vi "Weather Parse Test.vi"() -> ()   [LabVIEW 2020, in "CDM-Config.lvlib"] (continued)
                 ]\n                }\n            }\n        },\n        {\n            \"id\": \"https://api.weather.gov/alerts/urn:oid:2.49.0.1.840.0.415ec53db9f1e26240148abfa70e4c09e2d74678.012.1\",\n            \"type\": \"Feature\",\n            \"geometry\": null,\n            \"properties\": {\n                \"@id\": \"https://api.weather.gov/alerts/urn:oid:2.49.0.1.840.0.415ec53db9f1e26240148abfa70e4c09e2d74678.012.1\",\n                \"@type\": \"wx:Alert\",\n                \"id\": \"urn:oid:2.49.0.1.840.0.415ec53db9f1e26240148abfa70e4c09e2d74678.012.1\",\n                \"areaDesc\": \"Icy Cape to Cape Suckling out to 15 NM\",\n                \"geocode\": {\n                    \"SAME\": [\n                        \"058652\"\n                    ],\n                    \"UGC\": [\n                        \"PKZ652\"\n                    ]\n                },\n                \"affectedZones\": [\n                    \"https://api.weather.gov/zones/forecast/PKZ652\"\n                ],\n                \"references\": [],\n                \"sent\": \"2025-12-03T02:44:00-09:00\",\n                \"effective\": \"2025-12-03T02:44:00-09:00\",\n                \"onset\": \"2025-12-03T02:00:00-09:00\",\n                \"expires\": \"2025-12-03T20:45:00-09:00\",\n                \"ends\": \"2025-12-04T05:00:00-09:00\",\n                \"status\": \"Actual\",\n                \"messageType\": \"Alert\",\n                \"category\": \"Met\",\n                \"severity\": \"Minor\",\n                \"certainty\": \"Likely\",\n                \"urgency\": \"Expected\",\n                \"event\": \"Small Craft Advisory\",\n                \"sender\": \"w-nws.webmaster@noaa.gov\",\n                \"senderName\": \"NWS Juneau AK\",\n                \"headline\": \"Small Craft Advisory issued December 3 at 2:44AM AKST until December 4 at 5:00AM AKST by NWS Juneau AK\",\n                \"description\": \"Southeast Alaska Coastal Waters from Dixon Entrance to\\nCape Suckling out 100 NM\\n\\nWind forecasts reflect the predominant speed and direction\\nexpected. Seas forecasts represent the average of the highest\\none-third of the combined windwave and swell height.\\n\\n.TODAY...E wind 25 kt diminishing to 15 kt in the afternoon. Seas\\n12 ft. Rain.\\n.TONIGHT...Light winds becoming W 10 kt late. Seas 9 ft. SW\\nswell.\\n.THU...Light winds. Seas 8 ft. SW swell.\\n.THU NIGHT...E wind 10 kt. Seas 7 ft. SW swell.\\n.FRI...E wind 20 kt. Seas 7 ft.\\n.SAT...E gale to 35 kt. Seas 12 ft.\\n.SUN...E gale to 35 kt. Seas 15 ft.\",\n                \"instruction\": null,\n                \"response\": \"Avoid\",\n                \"parameters\": {\n                    \"AWIPSidentifier\": [\n                        \"CWFAEG\"\n                    ],\n                    \"WMOidentifier\": [\n                        \"FZAK52 PAJK 031144\"\n                    ],\n                    \"NWSheadline\": [\n                        \"SMALL CRAFT ADVISORY THROUGH LATE TONIGHT\"\n                    ],\n                    \"BLOCKCHANNEL\": [\n                        \"EAS\",\n                        \"NWEM\",\n                        \"CMAS\"\n                    ],\n                    \"VTEC\": [\n                        \"/O.NEW.PAJK.SC.Y.8602.251203T1100Z-251204T1400Z/\"\n                    ],\n                    \"eventEndingTime\": [\n                        \"2025-12-04T05:00:00-09:00\"\n                    ]\n                },\n                \"scope\": \"Public\",\n                \"code\": \"IPAWSv1.0\",\n                \"language\": \"en-US\",\n                \"web\": \"http://www.weather.gov\",\n                \"eventCode\": {\n                    \"SAME\": [\n                        \"NWS\"\n                    ],\n                    \"NationalWeatherService\": [\n                        \"SCY\"\n                    ]\n                }\n            }\n        },\n        {\n            \"id\": \"https://api.weather.gov/alerts/urn:oid:2.49.0.1.840.0.415ec53db9f1e26240148abfa70e4c09e2d74678.005.1\",\n            \"type\": \"Feature\",\n            \"geometry\": null,\n            \"properties\": {\n                \"@id\": \"https://api.weather.gov/alerts/urn:oid:2.49.0.1.840.0.415ec53db9f1e26240148abfa70e4c09e2d74678.005.1\",\n                \"@type\": \"wx:Alert\",\n                \"id\": \"urn:oid:2.49.0.1.840.0.415ec53db9f1e26240148abfa70e4c09e2d74678.005.1\",\n                \"areaDesc\": \"Cape Decision to Cape Edgecumbe from 15 to 80 NM\",\n                \"geocode\": {\n                    \"SAME\": [\n                        \"058662\"\n                    ],\n                    \"UGC\": [\n                        \"PKZ662\"\n                    ]\n                },\n                \"affectedZones\": [\n                    \"https://api.weather.gov/zones/forecast/PKZ662\"\n                ],\n                \"references\": [],\n                \"sent\": \"2025-12-03T02:44:00-09:00\",\n                \"effective\": \"2025-12-03T02:44:00-09:00\",\n                \"onset\": \"2025-12-03T02:00:00-09:00\",\n                \"expires\": \"2025-12-03T20:45:00-09:00\",\n                \"ends\": \"2025-12-04T05:00:00-09:00\",\n                \"status\": \"Actual\",\n                \"messageType\": \"Alert\",\n                \"category\": \"Met\",\n                \"severity\": \"Minor\",\n                \"certainty\": \"Likely\",\n                \"urgency\": \"Expected\",\n                \"event\": \"Small Craft Advisory\",\n                \"sender\": \"w-nws.webmaster@noaa.gov\",\n                \"senderName\": \"NWS Juneau AK\",\n                \"headline\": \"Small Craft Advisory issued December 3 at 2:44AM AKST until December 4 at 5:00AM AKST by NWS Juneau AK\",\n                \"description\": \"Southeast Alaska Coastal Waters from Dixon Entrance to\\nCape Suckling out 100 NM\\n\\nWind forecasts reflect the predominant speed and direction\\nexpected. Seas forecasts represent the average of the highest\\none-third of the combined windwave and swell height.\\n\\n.TODAY...S wind 20 kt becoming W in the afternoon. Seas 11 ft.\\n.TONIGHT...W wind 15 kt. Seas 10 ft.\\n.THU...W wind 10 kt becoming S in the afternoon. Seas 8 ft.\\n.THU NIGHT...SE wind 20 kt. Seas 9 ft.\\n.FRI...W wind 25 kt. Seas 14 ft.\\n.SAT...S wind 30 kt. Seas 16 ft.\\n.SUN...S gale to 35 kt. Seas 21 ft.\",\n                \"instruction\": null,\n                \"response\": \"Avoid\",\n                \"parameters\": {\n                    \"AWIPSidentifier\": [\n                        \"CWFAEG\"\n                    ],\n                    \"WMOidentifier\": [\n                        \"FZAK52 PAJK 031144\"\n                    ],\n                    \"NWSheadline\": [\n                        \"SMALL CRAFT ADVISORY THROUGH LATE TONIGHT\"\n                    ],\n                    \"BLOCKCHANNEL\": [\n                        \"EAS\",\n                        \"NWEM\",\n                        \"CMAS\"\n                    ],\n                    \"VTEC\": [\n                        \"/O.NEW.PAJK.SC.Y.8595.251203T1100Z-251204T1400Z/\"\n                    ],\n                    \"eventEndingTime\": [\n                        \"2025-12-04T05:00:00-09:00\"\n                    ]\n                },\n                \"scope\": \"Public\",\n                \"code\": \"IPAWSv1.0\",\n                \"language\": \"en-US\",\n                \"web\": \"http://www.weather.gov\",\n                \"eventCode\": {\n                    \"SAME\": [\n                        \"NWS\"\n                    ],\n                    \"NationalWeatherService\": [\n                        \"SCY\"\n                    ]\n                }\n            }\n        },\n        {\n            \"id\": \"https://api.weather.gov/alerts/urn:oid:2.49.0.1.840.0.415ec53db9f1e26240148abfa70e4c09e2d74678.009.1\",\n            \"type\": \"Feature\",\n            \"geometry\": null,\n            \"properties\": {\n                \"@id\": \"https://api.weather.gov/alerts/urn:oid:2.49.0.1.840.0.415ec53db9f1e26240148abfa70e4c09e2d74678.009.1\",\n                \"@type\": \"wx:Alert\",\n                \"id\": \"urn:oid:2.49.0.1.840.0.415ec53db9f1e26240148abfa70e4c09e2d74678.009.1\",\n                \"areaDesc\": \"Cape Spencer to Cape Fairweather from 15 to 85 NM\",\n                \"geocode\": {\n                    \"SAME\": [\n                        \"058664\"\n                    ],\n                    \"UGC\": [\n                        \"PKZ664\"\n                    ]\n                },\n                \"affectedZones\": [\n                    \"https://api.weather.gov/zones/forecast/PKZ664\"\n                ],\n                \"references\": [],\n                \"sent\": \"2025-12-03T02:44:00-09:00\",\n                \"effective\": \"2025-12-03T02:44:00-09:00\",\n                \"onset\": \"2025-12-03T02:00:00-09:00\",\n                \"expires\": \"2025-12-03T20:45:00-09:00\",\n                \"ends\": \"2025-12-04T05:00:00-09:00\",\n                \"status\": \"Actual\",\n                \"messageType\": \"Alert\",\n                \"category\": \"Met\",\n                \"severity\": \"Minor\",\n                \"certainty\": \"Likely\",\n                \"urgency\": \"Expected\",\n                \"event\": \"Small Craft Advisory\",\n                \"sender\": \"w-nws.webmaster@noaa.gov\",\n                \"senderName\": \"NWS Juneau AK\",\n                \"headline\": \"Small Craft Advisory issued December 3 at 2:44AM AKST until December 4 at 5:00AM AKST by NWS Juneau AK\",\n                \"description\": \"Southeast Alaska Coastal Waters from Dixon Entrance to\\nCape Suckling out 100 NM\\n\\nWind forecasts reflect the predominant speed and direction\\nexpected. Seas forecasts represent the average of the highest\\none-third of the combined windwave and swell height.\\n\\n.TODAY...S wind 25 kt becoming SW 15 kt in the afternoon. Seas\\n11 ft. SW swell.\\n.TONIGHT...W wind 20 kt. Seas 10 ft.\\n.THU...W wind 10 kt. Seas 9 ft.\\n.THU NIGHT...SE wind 20 kt. Seas 8 ft.\\n.FRI...SW wind 25 kt. Seas 9 ft.\\n.SAT...S gale to 35 kt. Seas 15 ft.\\n.SUN...S gale to 35 kt. Seas 18 ft.\",\n                \"instruction\": null,\n                \"response\": \"Avoid\",\n                \"parameters\": {\n                    \"AWIPSidentifier\": [\n                        \"CWFAEG\"\n                    ],\n                    \"WMOidentifier\": [\n                        \"FZAK52 PAJK 031144\"\n                    ],\n                    \"NWSheadline\": [\n                        \"SMALL CRAFT ADVISORY THROUGH LATE TONIGHT\"\n                    ],\n                    \"BLOCKCHANNEL\": [\n                        \"EAS\",\n                        \"NWEM\",\n                        \"CMAS\"\n                    ],\n                    \"VTEC\": [\n                        \"/O.NEW.PAJK.SC.Y.8599.251203T1100Z-251204T1400Z/\"\n                    ],\n                    \"eventEndingTime\": [\n                        \"2025-12-04T05:00:00-09:00\"\n                    ]\n                },\n                \"scope\": \"Public\",\n                \"code\": \"IPAWSv1.0\",\n                \"language\": \"en-US\",\n                \"web\": \"http://www.weather.gov\",\n                \"eventCode\": {\n                    \"SAME\": [\n                        \"NWS\"\n                    ],\n                    \"NationalWeatherService\": [\n                        \"SCY\"\n                    ]\n                }\n            }\n        },\n        {\n            \"id\": \"https://api.weather.gov/alerts/urn:oid:2.49.0.1.840.0.415ec53db9f1e26240148abfa70e4c09e2d74678.007.1\",\n            \"type\": \"Feature\",\n            \"geometry\": null,\n            \"properties\": {\n                \"@id\": \"https://api.weather.gov/alerts/urn:oid:2.49.0.1.840.0.415ec53db9f1e26240148abfa70e4c09e2d74678.007.1\",\n                \"@type\": \"wx:Alert\",\n                \"id\": \"urn:oid:2.49.0.1.840.0.415ec53db9f1e26240148abfa70e4c09e2d74678.007.1\",\n                \"areaDesc\": \"Cape Edgecumbe to Cape Spencer from 15 to 80 NM\",\n                \"geocode\": {\n                    \"SAME\": [\n                        \"058663\"\n                    ],\n                    \"UGC\": [\n                        \"PKZ663\"\n                    ]\n                },\n                \"affectedZones\": [\n                    \"https://api.weather.gov/zones/forecast/PKZ663\"\n                ],\n                \"references\": [],\n                \"sent\": \"2025-12-03T02:44:00-09:00\",\n                \"effective\": \"2025-12-03T02:44:00-09:00\",\n                \"onset\": \"2025-12-03T02:00:00-09:00\",\n                \"expires\": \"2025-12-03T20:45:00-09:00\",\n                \"ends\": \"2025-12-04T05:00:00-09:00\",\n                \"status\": \"Actual\",\n                \"messageType\": \"Alert\",\n                \"category\": \"Met\",\n                \"severity\": \"Minor\",\n                \"certainty\": \"Likely\",\n                \"urgency\": \"Expected\",\n                \"event\": \"Small Craft Advisory\",\n                \"sender\": \"w-nws.webmaster@noaa.gov\",\n                \"senderName\": \"NWS Juneau AK\",\n                \"headline\": \"Small Craft Advisory issued December 3 at 2:44AM AKST until December 4 at 5:00AM AKST by NWS Juneau AK\",\n                \"description\": \"Southeast Alaska Coastal Waters from Dixon Entrance to\\nCape Suckling out 100 NM\\n\\nWind forecasts reflect the predominant speed and direction\\nexpected. Seas forecasts represent the average of the highest\\none-third of the combined windwave and swell height.\\n\\n.TODAY...S wind 20 kt becoming W in the afternoon. Seas 11 ft.\\n.TONIGHT...W wind 20 kt. Seas 10 ft.\\n.THU...SW wind 10 kt. Seas 9 ft.\\n.THU NIGHT...SE wind 20 kt. Seas 9 ft.\\n.FRI...SW wind 20 kt. Seas 10 ft.\\n.SAT...S wind 30 kt. Seas 14 ft.\\n.SUN...S wind 30 kt. Seas 20 ft.\",\n                \"instruction\": null,\n                \"response\": \"Avoid\",\n                \"parameters\": {\n                    \"AWIPSidentifier\": [\n                        \"CWFAEG\"\n                    ],\n                    \"WMOidentifier\": [\n                        \"FZAK52 PAJK 031144\"\n                    ],\n                    \"NWSheadline\": [\n                        \"SMALL CRAFT ADVISORY THROUGH LATE TONIGHT\"\n                    ],\n                    \"BLOCKCHANNEL\": [\n                        \"EAS\",\n                        \"NWEM\",\n                        \"CMAS\"\n                    ],\n                    \"VTEC\": [\n                        \"/O.NEW.PAJK.SC.Y.8597.251203T1100Z-251204T1400Z/\"\n                    ],\n                    \"eventEndingTime\": [\n                        \"2025-12-04T05:00:00-09:00\"\n                    ]\n                },\n                \"scope\": \"Public\",\n                \"code\": \"IPAWSv1.0\",\n                \"language\": \"en-US\",\n                \"web\": \"http://www.weather.gov\",\n                \"eventCode\": {\n                    \"SAME\": [\n                        \"NWS\"\n                    ],\n                    \"NationalWeatherService\": [\n                        \"SCY\"\n                    ]\n                }\n            }\n        },\n        {\n            \"id\": \"https://api.weather.gov/alerts/urn:oid:2.49.0.1.840.0.415ec53db9f1e26240148abfa70e4c09e2d74678.008.1\",\n            \"type\": \"Feature\",\n            \"geometry\": null,\n            \"properties\": {\n                \"@id\": \"https://api.weather.gov/alerts/urn:oid:2.49.0.1.840.0.415ec53db9f1e26240148abfa70e4c09e2d74678.008.1\",\n                \"@type\": \"wx:Alert\",\n                \"id\": \"urn:oid:2.49.0.1.840.0.415ec53db9f1e26240148abfa70e4c09e2d74678.008.1\",\n                \"areaDesc\": \"Cape Spencer to Cape Fairweather out to 15 NM\",\n                \"geocode\": {\n                    \"SAME\": [\n                        \"058644\"\n                    ],\n                    \"UGC\": [\n                        \"PKZ644\"\n                    ]\n                },\n                \"affectedZones\": [\n                    \"https://api.weather.gov/zones/forecast/PKZ644\"\n                ],\n                \"references\": [],\n                \"sent\": \"2025-12-03T02:44:00-09:00\",\n                \"effective\": \"2025-12-03T02:44:00-09:00\",\n                \"onset\": \"2025-12-03T02:00:00-09:00\",\n                \"expires\": \"2025-12-03T20:45:00-09:00\",\n                \"ends\": \"2025-12-04T05:00:00-09:00\",\n                \"status\": \"Actual\",\n                \"messageType\": \"Alert\",\n                \"category\": \"Met\",\n                \"severity\": \"Minor\",\n                \"certainty\": \"Likely\",\n                \"urgency\": \"Expected\",\n                \"event\": \"Small Craft Advisory\",\n                \"sender\": \"w-nws.webmaster@noaa.gov\",\n                \"senderName\": \"NWS Juneau AK\",\n                \"headline\": \"Small Craft Advisory issued December 3 at 2:44AM AKST until December 4 at 5:00AM AKST by NWS Juneau AK\",\n                \"description\": \"Southeast Alaska Coastal Waters from Dixon Entrance to\\nCape Suckling out 100 NM\\n\\nWind forecasts reflect the predominant speed and direction\\nexpected. Seas forecasts represent the average of the highest\\none-third of the combined windwave and swell height.\\n\\n.TODAY...E wind 25 kt becoming SE 15 kt in the afternoon. Seas\\n11 ft. Rain.\\n.TONIGHT...W wind 15 kt. Seas 10 ft.\\n.THU...W wind 10 kt. Seas 9 ft.\\n.THU NIGHT...E wind 15 kt. Seas 8 ft.\\n.FRI...NE wind 25 kt. Seas 9 ft.\\n.SAT...S gale to 35 kt. Seas 14 ft.\\n.SUN...SE gale to 35 kt. Seas 17 ft.\",\n                \"instruction\": null,\n                \"response\": \"Avoid\",\n                \"parameters\": {\n                    \"AWIPSidentifier\": [\n                        \"CWFAEG\"\n                    ],\n                    \"WMOidentifier\": [\n                        \"FZAK52 PAJK 031144\"\n                    ],\n                    \"NWSheadline\": [\n                        \"SMALL CRAFT ADVISORY THROUGH LATE TONIGHT\"\n                    ],\n                    \"BLOCKCHANNEL\": [\n                        \"EAS\",\n                        \"NWEM\",\n                        \"CMAS\"\n                    ],\n                    \"VTEC\": [\n                        \"/O.NEW.PAJK.SC.Y.8598.251203T1100Z-251204T1400Z/\"\n                    ],\n                    \"eventEndingTime\": [\n                        \"2025-12-04T05:00:00-09:00\"\n                    ]\n                },\n                \"scope\": \"Public\",\n                \"code\": \"IPAWSv1.0\",\n                \"language\": \"en-US\",\n                \"web\": \"http://www.weather.gov\",\n                \"eventCode\": {\n                    \"SAME\": [\n                        \"NWS\"\n                    ],\n                    \"NationalWeatherService\": [\n                        \"SCY\"\n                    ]\n                }\n            }\n        },\n        {\n            \"id\": \"https://api.weather.gov/alerts/urn:oid:2.49.0.1.840.0.415ec53db9f1e26240148abfa70e4c09e2d74678.006.1\",\n            \"type\": \"Feature\",\n            \"geometry\": null,\n            \"properties\": {\n                \"@id\": \"https://api.weather.gov/alerts/urn:oid:2.49.0.1.840.0.415ec53db9f1e26240148abfa70e4c09e2d74678.006.1\",\n                \"@type\": \"wx:Alert\",\n                \"id\": \"urn:oid:2.49.0.1.840.0.415ec53db9f1e26240148abfa70e4c09e2d74678.006.1\",\n                \"areaDesc\": \"Cape Edgecumbe to Cape Spencer out to 15 NM\",\n                \"geocode\": {\n                    \"SAME\": [\n                        \"058643\"\n                    ],\n                    \"UGC\": [\n                        \"PKZ643\"\n                    ]\n                },\n                \"affectedZones\": [\n                    \"https://api.weather.gov/zones/forecast/PKZ643\"\n                ],\n                \"references\": [],\n                \"sent\": \"2025-12-03T02:44:00-09:00\",\n                \"effective\": \"2025-12-03T02:44:00-09:00\",\n                \"onset\": \"2025-12-03T02:00:00-09:00\",\n                \"expires\": \"2025-12-03T20:45:00-09:00\",\n                \"ends\": \"2025-12-04T05:00:00-09:00\",\n                \"status\": \"Actual\",\n                \"messageType\": \"Alert\",\n                \"category\": \"Met\",\n                \"severity\": \"Minor\",\n                \"certainty\": \"Likely\",\n                \"urgency\": \"Expected\",\n                \"event\": \"Small Craft Advisory\",\n                \"sender\": \"w-nws.webmaster@noaa.gov\",\n                \"senderName\": \"NWS Juneau AK\",\n                \"headline\": \"Small Craft Advisory issued December 3 at 2:44AM AKST until December 4 at 5:00AM AKST by NWS Juneau AK\",\n                \"description\": \"Southeast Alaska Coastal Waters from Dixon Entrance to\\nCape Suckling out 100 NM\\n\\nWind forecasts reflect the predominant speed and direction\\nexpected. Seas forecasts represent the average of the highest\\none-third of the combined windwave and swell height.\\n\\n.TODAY...SE wind 25 kt becoming SW 15 kt in the afternoon. Seas\\n11 ft. Rain early in the morning.\\n.TONIGHT...W wind 15 kt. Seas 10 ft.\\n.THU...SW wind 10 kt. Seas 9 ft.\\n.THU NIGHT...E wind 15 kt. Seas 8 ft.\\n.FRI...NE wind 20 kt. Seas 10 ft.\\n.SAT...S wind 30 kt. Seas 13 ft.\\n.SUN...S wind 30 kt. Seas 17 ft.\",\n                \"instruction\": null,\n                \"response\": \"Avoid\",\n                \"parameters\": {\n                    \"AWIPSidentifier\": [\n                        \"CWFAEG\"\n                    ],\n                    \"WMOidentifier\": [\n                        \"FZAK52 PAJK 031144\"\n                    ],\n                    \"NWSheadline\": [\n                        \"SMALL CRAFT ADVISORY THROUGH LATE TONIGHT\"\n                    ],\n                    \"BLOCKCHANNEL\": [\n                        \"EAS\",\n                        \"NWEM\",\n                        \"CMAS\"\n                    ],\n                    \"VTEC\": [\n                        \"/O.NEW.PAJK.SC.Y.8596.251203T1100Z-251204T1400Z/\"\n                    ],\n                    \"eventEndingTime\": [\n                        \"2025-12-04T05:00:00-09:00\"\n                    ]\n                },\n                \"scope\": \"Public\",\n                \"code\": \"IPAWSv1.0\",\n                \"language\": \"en-US\",\n                \"web\": \"http://www.weather.gov\",\n                \"eventCode\": {\n                    \"SAME\": [\n                        \"NWS\"\n                    ],\n                    \"NationalWeatherService\": [\n                        \"SCY\"\n                    ]\n                }\n            }\n        },\n        {\n            \"id\": \"https://api.weather.gov/alerts/urn:oid:2.49.0.1.840.0.415ec53db9f1e26240148abfa70e4c09e2d74678.010.1\",\n            \"type\": \"Feature\",\n            \"geometry\": null,\n            \"properties\": {\n                \"@id\": \"https://api.weather.gov/alerts/urn:oid:2.49.0.1.840.0.415ec53db9f1e26240148abfa70e4c09e2d74678.010.1\",\n                \"@type\": \"wx:Alert\",\n                \"id\": \"urn:oid:2.49.0.1.840.0.415ec53db9f1e26240148abfa70e4c09e2d74678.010.1\",\n                \"areaDesc\": \"Cape Fairweather to Icy Cape out to 15 NM\",\n                \"geocode\": {\n                    \"SAME\": [\n                        \"058651\"\n                    ],\n                    \"UGC\": [\n                        \"PKZ651\"\n                    ]\n                },\n                \"affectedZones\": [\n                    \"https://api.weather.gov/zones/forecast/PKZ651\"\n                ],\n                \"references\": [],\n                \"sent\": \"2025-12-03T02:44:00-09:00\",\n                \"effective\": \"2025-12-03T02:44:00-09:00\",\n                \"onset\": \"2025-12-03T02:00:00-09:00\",\n                \"expires\": \"2025-12-03T20:45:00-09:00\",\n                \"ends\": \"2025-12-04T05:00:00-09:00\",\n                \"status\": \"Actual\",\n                \"messageType\": \"Alert\",\n                \"category\": \"Met\",\n                \"severity\": \"Minor\",\n                \"certainty\": \"Likely\",\n                \"urgency\": \"Expected\",\n                \"event\": \"Small Craft Advisory\",\n                \"sender\": \"w-nws.webmaster@noaa.gov\",\n                \"senderName\": \"NWS Juneau AK\",\n                \"headline\": \"Small Craft Advisory issued December 3 at 2:44AM AKST until December 4 at 5:00AM AKST by NWS Juneau AK\",\n                \"description\": \"Southeast Alaska Coastal Waters from Dixon Entrance to\\nCape Suckling out 100 NM\\n\\nWind forecasts reflect the predominant speed and direction\\nexpected. Seas forecasts represent the average of the highest\\none-third of the combined windwave and swell height.\\n\\n.TODAY...SE wind 25 kt becoming SW 15 kt in the afternoon. Seas\\n11 ft. Rain.\\n.TONIGHT...W wind 10 kt. Seas 10 ft.\\n.THU...Light winds becoming E 10 kt in the afternoon. Seas\\n8 ft. SW swell.\\n.THU NIGHT...E wind 10 kt. Seas 7 ft. SW swell.\\n.FRI...E wind 25 kt. Seas 9 ft.\\n.SAT...E gale to 35 kt. Seas 14 ft.\\n.SUN...E gale to 35 kt. Seas 16 ft.\",\n                \"instruction\": null,\n                \"response\": \"Avoid\",\n                \"parameters\": {\n                    \"AWIPSidentifier\": [\n                        \"CWFAEG\"\n                    ],\n                    \"WMOidentifier\": [\n                        \"FZAK52 PAJK 031144\"\n                    ],\n                    \"NWSheadline\": [\n                        \"SMALL CRAFT ADVISORY THROUGH LATE TONIGHT\"\n                    ],\n                    \"BLOCKCHANNEL\": [\n                        \"EAS\",\n                        \"NWEM\",\n                        \"CMAS\"\n                    ],\n                    \"VTEC\": [\n                        \"/O.NEW.PAJK.SC.Y.8600.251203T1100Z-251204T1400Z/\"\n                    ],\n                    \"eventEndingTime\": [\n                        \"2025-12-04T05:00:00-09:00\"\n                    ]\n                },\n                \"scope\": \"Public\",\n                \"code\": \"IPAWSv1.0\",\n                \"language\": \"en-US\",\n                \"web\": \"http://www.weather.gov\",\n                \"eventCode\": {\n                    \"SAME\": [\n                        \"NWS\"\n                    ],\n                    \"NationalWeatherService\": [\n                        \"SCY\"\n                    ]\n                }\n            }\n        },\n        {\n            \"id\": \"https://api.weather.gov/alerts/urn:oid:2.49.0.1.840.0.415ec53db9f1e26240148abfa70e4c09e2d74678.002.1\",\n            \"type\": \"Feature\",\n            \"geometry\": null,\n            \"properties\": {\n                \"@id\": \"https://api.weather.gov/alerts/urn:oid:2.49.0.1.840.0.415ec53db9f1e26240148abfa70e4c09e2d74678.002.1\",\n                \"@type\": \"wx:Alert\",\n                \"id\": \"urn:oid:2.49.0.1.840.0.415ec53db9f1e26240148abfa70e4c09e2d74678.002.1\",\n                \"areaDesc\": \"Dixon Entrance to Cape Decision out to 15 NM\",\n                \"geocode\": {\n                    \"SAME\": [\n                        \"058641\"\n                    ],\n                    \"UGC\": [\n                        \"PKZ641\"\n                    ]\n                },\n                \"affectedZones\": [\n                    \"https://api.weather.gov/zones/forecast/PKZ641\"\n                ],\n                \"references\": [],\n                \"sent\": \"2025-12-03T02:44:00-09:00\",\n                \"effective\": \"2025-12-03T02:44:00-09:00\",\n                \"onset\": \"2025-12-03T02:00:00-09:00\",\n                \"expires\": \"2025-12-03T20:45:00-09:00\",\n                \"ends\": \"2025-12-04T05:00:00-09:00\",\n                \"status\": \"Actual\",\n                \"messageType\": \"Alert\",\n                \"category\": \"Met\",\n                \"severity\": \"Minor\",\n                \"certainty\": \"Likely\",\n                \"urgency\": \"Expected\",\n                \"event\": \"Small Craft Advisory\",\n                \"sender\": \"w-nws.webmaster@noaa.gov\",\n                \"senderName\": \"NWS Juneau AK\",\n                \"headline\": \"Small Craft Advisory issued December 3 at 2:44AM AKST until December 4 at 5:00AM AKST by NWS Juneau AK\",\n                \"description\": \"Southeast Alaska Coastal Waters from Dixon Entrance to\\nCape Suckling out 100 NM\\n\\nWind forecasts reflect the predominant speed and direction\\nexpected. Seas forecasts represent the average of the highest\\none-third of the combined windwave and swell height.\\n\\n.TODAY...SE wind 25 kt becoming W 15 kt in the afternoon. Seas\\n11 ft. Rain early in the morning.\\n.TONIGHT...W wind 10 kt. Seas 10 ft.\\n.THU...W wind 10 kt becoming SE in the afternoon. Seas 8 ft.\\nSW swell.\\n.THU NIGHT...SE wind 20 kt. Seas 9 ft. Rain.\\n.FRI...W wind 25 kt. Seas 15 ft.\\n.SAT...S wind 30 kt. Seas 15 ft.\\n.SUN...S gale to 40 kt. Seas 20 ft.\",\n                \"instruction\": null,\n                \"response\": \"Avoid\",\n                \"parameters\": {\n                    \"AWIPSidentifier\": [\n                        \"CWFAEG\"\n                    ],\n                    \"WMOidentifier\": [\n                        \"FZAK52 PAJK 031144\"\n                    ],\n                    \"NWSheadline\": [\n                        \"SMALL CRAFT ADVISORY THROUGH LATE TONIGHT\"\n                    ],\n                    \"BLOCKCHANNEL\": [\n                        \"EAS\",\n                        \"NWEM\",\n                        \"CMAS\"\n                    ],\n                    \"VTEC\": [\n                        \"/O.NEW.PAJK.SC.Y.8592.251203T1100Z-251204T1400Z/\"\n                    ],\n                    \"eventEndingTime\": [\n                        \"2025-12-04T05:00:00-09:00\"\n                    ]\n                },\n                \"scope\": \"Public\",\n                \"code\": \"IPAWSv1.0\",\n                \"language\": \"en-US\",\n                \"web\": \"http://www.weather.gov\",\n                \"eventCode\": {\n                    \"SAME\": [\n                        \"NWS\"\n                    ],\n                    \"NationalWeatherService\": [\n                        \"SCY\"\n                    ]\n                }\n            }\n        },\n        {\n            \"id\": \"https://api.weather.gov/alerts/urn:oid:2.49.0.1.840.0.415ec53db9f1e26240148abfa70e4c09e2d74678.004.1\",\n            \"type\": \"Feature\",\n            \"geometry\": null,\n            \"properties\": {\n                \"@id\": \"https://api.weather.gov/alerts/urn:oid:2.49.0.1.840.0.415ec53db9f1e26240148abfa70e4c09e2d74678.004.1\",\n                \"@type\": \"wx:Alert\",\n                \"id\": \"urn:oid:2.49.0.1.840.0.415ec53db9f1e26240148abfa70e4c09e2d74678.004.1\",\n                \"areaDesc\": \"Cape Decision to Cape Edgecumbe out to 15 NM\",\n                \"geocode\": {\n                    \"SAME\": [\n                        \"058642\"\n                    ],\n                    \"UGC\": [\n                        \"PKZ642\"\n                    ]\n                },\n                \"affectedZones\": [\n                    \"https://api.weather.gov/zones/forecast/PKZ642\"\n                ],\n                \"references\": [],\n                \"sent\": \"2025-12-03T02:44:00-09:00\",\n                \"effective\": \"2025-12-03T02:44:00-09:00\",\n                \"onset\": \"2025-12-03T02:00:00-09:00\",\n                \"expires\": \"2025-12-03T20:45:00-09:00\",\n                \"ends\": \"2025-12-04T05:00:00-09:00\",\n                \"status\": \"Actual\",\n                \"messageType\": \"Alert\",\n                \"category\": \"Met\",\n                \"severity\": \"Minor\",\n                \"certainty\": \"Likely\",\n                \"urgency\": \"Expected\",\n                \"event\": \"Small Craft Advisory\",\n                \"sender\": \"w-nws.webmaster@noaa.gov\",\n                \"senderName\": \"NWS Juneau AK\",\n                \"headline\": \"Small Craft Advisory issued December 3 at 2:44AM AKST until December 4 at 5:00AM AKST by NWS Juneau AK\",\n                \"description\": \"Southeast Alaska Coastal Waters from Dixon Entrance to\\nCape Suckling out 100 NM\\n\\nWind forecasts reflect the predominant speed and direction\\nexpected. Seas forecasts represent the average of the highest\\none-third of the combined windwave and swell height.\\n\\n.TODAY...SE wind 25 kt becoming W 15 kt in the afternoon. Seas\\n11 ft. Rain early in the morning.\\n.TONIGHT...W wind 15 kt. Seas 10 ft.\\n.THU...W wind 10 kt becoming S in the afternoon. Seas 8 ft.\\n.THU NIGHT...E wind 20 kt. Seas 9 ft.\\n.FRI...W wind 20 kt. Seas 13 ft.\\n.SAT...S wind 30 kt. Seas 15 ft.\\n.SUN...S gale to 35 kt. Seas 20 ft.\",\n                \"instruction\": null,\n                \"response\": \"Avoid\",\n                \"parameters\": {\n                    \"AWIPSidentifier\": [\n                        \"CWFAEG\"\n                    ],\n                    \"WMOidentifier\": [\n                        \"FZAK52 PAJK 031144\"\n                    ],\n                    \"NWSheadline\": [\n                        \"SMALL CRAFT ADVISORY THROUGH LATE TONIGHT\"\n                    ],\n                    \"BLOCKCHANNEL\": [\n                        \"EAS\",\n                        \"NWEM\",\n                        \"CMAS\"\n                    ],\n                    \"VTEC\": [\n                        \"/O.NEW.PAJK.SC.Y.8594.251203T1100Z-251204T1400Z/\"\n                    ],\n                    \"eventEndingTime\": [\n                        \"2025-12-04T05:00:00-09:00\"\n                    ]\n                },\n                \"scope\": \"Public\",\n                \"code\": \"IPAWSv1.0\",\n                \"language\": \"en-US\",\n                \"web\": \"http://www.weather.gov\",\n                \"eventCode\": {\n                    \"SAME\": [\n                        \"NWS\"\n                    ],\n                    \"NationalWeatherService\": [\n                        \"SCY\"\n                    ]\n                }\n            }\n        },\n        {\n            \"id\": \"https://api.weather.gov/alerts/urn:oid:2.49.0.1.840.0.415ec53db9f1e26240148abfa70e4c09e2d74678.003.1\",\n            \"type\": \"Feature\",\n            \"geometry\": null,\n            \"properties\": {\n                \"@id\": \"https://api.weather.gov/alerts/urn:oid:2.49.0.1.840.0.415ec53db9f1e26240148abfa70e4c09e2d74678.003.1\",\n                \"@type\": \"wx:Alert\",\n                \"id\": \"urn:oid:2.49.0.1.840.0.415ec53db9f1e26240148abfa70e4c09e2d74678.003.1\",\n                \"areaDesc\": \"Dixon Entrance to Cape Decision from 15 to 90 NM\",\n                \"geocode\": {\n                    \"SAME\": [\n                        \"058661\"\n                    ],\n                    \"UGC\": [\n                        \"PKZ661\"\n                    ]\n                },\n                \"affectedZones\": [\n                    \"https://api.weather.gov/zones/forecast/PKZ661\"\n                ],\n                \"references\": [],\n                \"sent\": \"2025-12-03T02:44:00-09:00\",\n                \"effective\": \"2025-12-03T02:44:00-09:00\",\n                \"onset\": \"2025-12-03T02:00:00-09:00\",\n                \"expires\": \"2025-12-03T20:45:00-09:00\",\n                \"ends\": \"2025-12-04T05:00:00-09:00\",\n                \"status\": \"Actual\",\n                \"messageType\": \"Alert\",\n                \"category\": \"Met\",\n                \"severity\": \"Minor\",\n                \"certainty\": \"Likely\",\n                \"urgency\": \"Expected\",\n                \"event\": \"Small Craft Advisory\",\n                \"sender\": \"w-nws.webmaster@noaa.gov\",\n                \"senderName\": \"NWS Juneau AK\",\n                \"headline\": \"Small Craft Advisory issued December 3 at 2:44AM AKST until December 4 at 5:00AM AKST by NWS Juneau AK\",\n                \"description\": \"Southeast Alaska Coastal Waters from Dixon Entrance to\\nCape Suckling out 100 NM\\n\\nWind forecasts reflect the predominant speed and direction\\nexpected. Seas forecasts represent the average of the highest\\none-third of the combined windwave and swell height.\\n\\n.TODAY...SW wind 20 kt becoming W in the afternoon. Seas 11 ft.\\nRain early in the morning.\\n.TONIGHT...W wind 15 kt. Seas 10 ft.\\n.THU...W wind 10 kt becoming SE in the afternoon. Seas 8 ft.\\nSW swell.\\n.THU NIGHT...SE wind 25 kt. Seas 9 ft. Rain.\\n.FRI...W wind 25 kt. Seas 17 ft.\\n.SAT...SW wind 30 kt. Seas 16 ft.\\n.SUN...SW gale to 35 kt. Seas 22 ft.\",\n                \"instruction\": null,\n                \"response\": \"Avoid\",\n                \"parameters\": {\n                    \"AWIPSidentifier\": [\n                        \"CWFAEG\"\n                    ],\n                    \"WMOidentifier\": [\n                        \"FZAK52 PAJK 031144\"\n                    ],\n                    \"NWSheadline\": [\n                        \"SMALL CRAFT ADVISORY THROUGH LATE TONIGHT\"\n                    ],\n                    \"BLOCKCHANNEL\": [\n                        \"EAS\",\n                        \"NWEM\",\n                        \"CMAS\"\n                    ],\n                    \"VTEC\": [\n                        \"/O.NEW.PAJK.SC.Y.8593.251203T1100Z-251204T1400Z/\"\n                    ],\n                    \"eventEndingTime\": [\n                        \"2025-12-04T05:00:00-09:00\"\n                    ]\n                },\n                \"scope\": \"Public\",\n                \"code\": \"IPAWSv1.0\",\n                \"language\": \"en-US\",\n                \"web\": \"http://www.weather.gov\",\n                \"eventCode\": {\n                    \"SAME\": [\n                        \"NWS\"\n                    ],\n                    \"NationalWeatherService\": [\n                        \"SCY\"\n                    ]\n                }\n            }\n        },\n        {\n            \"id\": \"https://api.weather.gov/alerts/urn:oid:2.49.0.1.840.0.415ec53db9f1e26240148abfa70e4c09e2d74678.013.1\",\n            \"type\": \"Feature\",\n            \"geometry\": null,\n            \"properties\": {\n                \"@id\": \"https://api.weather.gov/alerts/urn:oid:2.49.0.1.840.0.415ec53db9f1e26240148abfa70e4c09e2d74678.013.1\",\n                \"@type\": \"wx:Alert\",\n                \"id\": \"urn:oid:2.49.0.1.840.0.415ec53db9f1e26240148abfa70e4c09e2d74678.013.1\",\n                \"areaDesc\": \"Icy Cape to Cape Suckling from 15 to 80 NM\",\n                \"geocode\": {\n                    \"SAME\": [\n                        \"058672\"\n                    ],\n                    \"UGC\": [\n                        \"PKZ672\"\n                    ]\n                },\n                \"affectedZones\": [\n                    \"https://api.weather.gov/zones/forecast/PKZ672\"\n                ],\n                \"references\": [],\n                \"sent\": \"2025-12-03T02:44:00-09:00\",\n                \"effective\": \"2025-12-03T02:44:00-09:00\",\n                \"onset\": \"2025-12-03T02:00:00-09:00\",\n                \"expires\": \"2025-12-03T20:45:00-09:00\",\n                \"ends\": \"2025-12-04T05:00:00-09:00\",\n                \"status\": \"Actual\",\n                \"messageType\": \"Alert\",\n                \"category\": \"Met\",\n                \"severity\": \"Minor\",\n                \"certainty\": \"Likely\",\n                \"urgency\": \"Expected\",\n                \"event\": \"Small Craft Advisory\",\n                \"sender\": \"w-nws.webmaster@noaa.gov\",\n                \"senderName\": \"NWS Juneau AK\",\n                \"headline\": \"Small Craft Advisory issued December 3 at 2:44AM AKST until December 4 at 5:00AM AKST by NWS Juneau AK\",\n                \"description\": \"Southeast Alaska Coastal Waters from Dixon Entrance to\\nCape Suckling out 100 NM\\n\\nWind forecasts reflect the predominant speed and direction\\nexpected. Seas forecasts represent the average of the highest\\none-third of the combined windwave and swell height.\\n\\n.TODAY...E wind 25 kt becoming SW 15 kt in the afternoon. Seas\\n12 ft.\\n.TONIGHT...W wind 15 kt. Seas 10 ft.\\n.THU...SW wind 10 kt. Seas 8 ft. SW swell.\\n.THU NIGHT...E wind 10 kt. Seas 8 ft.\\n.FRI...S wind 20 kt. Seas 8 ft.\\n.SAT...SE wind 30 kt. Seas 13 ft.\\n.SUN...SE wind 30 kt. Seas 16 ft.\",\n                \"instruction\": null,\n                \"response\": \"Avoid\",\n                \"parameters\": {\n                    \"AWIPSidentifier\": [\n                        \"CWFAEG\"\n                    ],\n                    \"WMOidentifier\": [\n                        \"FZAK52 PAJK 031144\"\n                    ],\n                    \"NWSheadline\": [\n                        \"SMALL CRAFT ADVISORY THROUGH LATE TONIGHT\"\n                    ],\n                    \"BLOCKCHANNEL\": [\n                        \"EAS\",\n                        \"NWEM\",\n                        \"CMAS\"\n                    ],\n                    \"VTEC\": [\n                        \"/O.NEW.PAJK.SC.Y.8603.251203T1100Z-251204T1400Z/\"\n                    ],\n                    \"eventEndingTime\": [\n                        \"2025-12-04T05:00:00-09:00\"\n                    ]\n                },\n                \"scope\": \"Public\",\n                \"code\": \"IPAWSv1.0\",\n                \"language\": \"en-US\",\n                \"web\": \"http://www.weather.gov\",\n                \"eventCode\": {\n                    \"SAME\": [\n                        \"NWS\"\n                    ],\n                    \"NationalWeatherService\": [\n                        \"SCY\"\n                    ]\n                }\n            }\n        },\n        {\n            \"id\": \"https://api.weather.gov/alerts/urn:oid:2.49.0.1.840.0.415ec53db9f1e26240148abfa70e4c09e2d74678.011.1\",\n            \"type\": \"Feature\",\n            \"geometry\": null,\n            \"properties\": {\n                \"@id\": \"https://api.weather.gov/alerts/urn:oid:2.49.0.1.840.0.415ec53db9f1e26240148abfa70e4c09e2d74678.011.1\",\n                \"@type\": \"wx:Alert\",\n                \"id\": \"urn:oid:2.49.0.1.840.0.415ec53db9f1e26240148abfa70e4c09e2d74678.011.1\",\n                \"areaDesc\": \"Cape Fairweather to Icy Cape from 15 to 80 NM\",\n                \"geocode\": {\n                    \"SAME\": [\n                        \"058671\"\n                    ],\n                    \"UGC\": [\n                        \"PKZ671\"\n                    ]\n                },\n                \"affectedZones\": [\n                    \"https://api.weather.gov/zones/forecast/PKZ671\"\n                ],\n                \"references\": [],\n                \"sent\": \"2025-12-03T02:44:00-09:00\",\n                \"effective\": \"2025-12-03T02:44:00-09:00\",\n                \"onset\": \"2025-12-03T02:00:00-09:00\",\n                \"expires\": \"2025-12-03T20:45:00-09:00\",\n                \"ends\": \"2025-12-04T05:00:00-09:00\",\n                \"status\": \"Actual\",\n                \"messageType\": \"Alert\",\n                \"category\": \"Met\",\n                \"severity\": \"Minor\",\n                \"certainty\": \"Likely\",\n                \"urgency\": \"Expected\",\n                \"event\": \"Small Craft Advisory\",\n                \"sender\": \"w-nws.webmaster@noaa.gov\",\n                \"senderName\": \"NWS Juneau AK\",\n                \"headline\": \"Small Craft Advisory issued December 3 at 2:44AM AKST until December 4 at 5:00AM AKST by NWS Juneau AK\",\n                \"description\": \"Southeast Alaska Coastal Waters from Dixon Entrance to\\nCape Suckling out 100 NM\\n\\nWind forecasts reflect the predominant speed and direction\\nexpected. Seas forecasts represent the average of the highest\\none-third of the combined windwave and swell height.\\n\\n.TODAY...S wind 25 kt becoming SW 15 kt in the afternoon. Seas\\n11 ft. SW swell. Rain early in the morning.\\n.TONIGHT...W wind 15 kt. Seas 10 ft.\\n.THU...SW wind 10 kt. Seas 9 ft.\\n.THU NIGHT...E wind 15 kt. Seas 8 ft.\\n.FRI...S wind 25 kt. Seas 9 ft.\\n.SAT...S gale to 35 kt. Seas 14 ft.\\n.SUN...SE gale to 35 kt. Seas 17 ft.\",\n                \"instruction\": null,\n                \"response\": \"Avoid\",\n                \"parameters\": {\n                    \"AWIPSidentifier\": [\n                        \"CWFAEG\"\n                    ],\n                    \"WMOidentifier\": [\n                        \"FZAK52 PAJK 031144\"\n                    ],\n                    \"NWSheadline\": [\n                        \"SMALL CRAFT ADVISORY THROUGH LATE TONIGHT\"\n                    ],\n                    \"BLOCKCHANNEL\": [\n                        \"EAS\",\n                        \"NWEM\",\n                        \"CMAS\"\n                    ],\n                    \"VTEC\": [\n                        \"/O.NEW.PAJK.SC.Y.8601.251203T1100Z-251204T1400Z/\"\n                    ],\n                    \"eventEndingTime\": [\n                        \"2025-12-04T05:00:00-09:00\"\n                    ]\n                },\n                \"scope\": \"Public\",\n                \"code\": \"IPAWSv1.0\",\n                \"language\": \"en-US\",\n                \"web\": \"http://www.weather.gov\",\n                \"eventCode\": {\n                    \"SAME\": [\n                        \"NWS\"\n                    ],\n                    \"NationalWeatherService\": [\n                        \"SCY\"\n                    ]\n                }\n            }\n        },\n        {\n            \"id\": \"https://api.weather.gov/alerts/urn:oid:2.49.0.1.840.0.94e4e19bc8eeb6087cc59420c6880e7d952ab5fe.006.1\",\n            \"type\": \"Feature\",\n            \"geometry\": null,\n            \"properties\": {\n                \"@id\": \"https://api.weather.gov/alerts/urn:oid:2.49.0.1.840.0.94e4e19bc8eeb6087cc59420c6880e7d952ab5fe.006.1\",\n                \"@type\": \"wx:Alert\",\n                \"id\": \"urn:oid:2.49.0.1.840.0.94e4e19bc8eeb6087cc59420c6880e7d952ab5fe.006.1\",\n                \"areaDesc\": \"Cross Sound\",\n                \"geocode\": {\n                    \"SAME\": [\n                        \"058022\"\n                    ],\n                    \"UGC\": [\n                        \"PKZ022\"\n                    ]\n                },\n                \"affectedZones\": [\n                    \"https://api.weather.gov/zones/forecast/PKZ022\"\n                ],\n                \"references\": [],\n                \"sent\": \"2025-12-03T02:44:00-09:00\",\n                \"effective\": \"2025-12-03T02:44:00-09:00\",\n                \"onset\": \"2025-12-03T02:00:00-09:00\",\n                \"expires\": \"2025-12-03T18:45:00-09:00\",\n                \"ends\": \"2025-12-04T05:00:00-09:00\",\n                \"status\": \"Actual\",\n                \"messageType\": \"Alert\",\n                \"category\": \"Met\",\n                \"severity\": \"Minor\",\n                \"certainty\": \"Likely\",\n                \"urgency\": \"Expected\",\n                \"event\": \"Small Craft Advisory\",\n                \"sender\": \"w-nws.webmaster@noaa.gov\",\n                \"senderName\": \"NWS Juneau AK\",\n                \"headline\": \"Small Craft Advisory issued December 3 at 2:44AM AKST until December 4 at 5:00AM AKST by NWS Juneau AK\",\n                \"description\": \"Southeast Alaska Inside Waters from Dixon Entrance to Skagway\\n\\nWind forecasts reflect the predominant speed and direction\\nexpected. Sea forecasts represent the average of the highest\\none-third of the combined windwave and swell height.\\n\\n.TODAY...E wind 15 kt becoming SW in the afternoon. Seas 9 ft.\\nRain.\\n.TONIGHT...SW wind 20 kt. Seas 8 ft. S swell. Rain in the\\nevening.\\n.THU...SW wind 10 kt. Seas 8 ft. Rain in the afternoon.\\n.THU NIGHT...NE wind 10 kt. Seas 7 ft. Rain.\\n.FRI...NE wind 15 kt. Seas 7 ft.\\n.SAT...S wind 25 kt. Seas 10 ft.\\n.SUN...E wind 30 kt. Seas 12 ft.\",\n                \"instruction\": null,\n                \"response\": \"Avoid\",\n                \"parameters\": {\n                    \"AWIPSidentifier\": [\n                        \"CWFAJK\"\n                    ],\n                    \"WMOidentifier\": [\n                        \"FZAK51 PAJK 031144\"\n                    ],\n                    \"NWSheadline\": [\n                        \"SMALL CRAFT ADVISORY THROUGH LATE TONIGHT\"\n                    ],\n                    \"BLOCKCHANNEL\": [\n                        \"EAS\",\n                        \"NWEM\",\n                        \"CMAS\"\n                    ],\n                    \"VTEC\": [\n                        \"/O.NEW.PAJK.SC.Y.7964.251203T1100Z-251204T1400Z/\"\n                    ],\n                    \"eventEndingTime\": [\n                        \"2025-12-04T05:00:00-09:00\"\n                    ]\n                },\n                \"scope\": \"Public\",\n                \"code\": \"IPAWSv1.0\",\n                \"language\": \"en-US\",\n                \"web\": \"http://www.weather.gov\",\n                \"eventCode\": {\n                    \"SAME\": [\n                        \"NWS\"\n                    ],\n                    \"NationalWeatherService\": [\n                        \"SCY\"\n                    ]\n                }\n            }\n        },\n        {\n            \"id\": \"https://api.weather.gov/alerts/urn:oid:2.49.0.1.840.0.4ff5fe1b1d40c5518c7c751190066b30fc728126.001.1\",\n            \"type\": \"Feature\",\n            \"geometry\": null,\n            \"properties\": {\n                \"@id\": \"https://api.weather.gov/alerts/urn:oid:2.49.0.1.840.0.4ff5fe1b1d40c5518c7c751190066b30fc728126.001.1\",\n                \"@type\": \"wx:Alert\",\n                \"id\": \"urn:oid:2.49.0.1.840.0.4ff5fe1b1d40c5518c7c751190066b30fc728126.001.1\",\n                \"areaDesc\": \"Yakutat Bay\",\n                \"geocode\": {\n                    \"SAME\": [\n                        \"058053\"\n                    ],\n                    \"UGC\": [\n                        \"PKZ053\"\n                    ]\n                },\n                \"affectedZones\": [\n                    \"https://api.weather.gov/zones/forecast/PKZ053\"\n                ],\n                \"references\": [],\n                \"sent\": \"2025-12-03T02:44:00-09:00\",\n                \"effective\": \"2025-12-03T02:44:00-09:00\",\n                \"onset\": \"2025-12-03T02:00:00-09:00\",\n                \"expires\": \"2025-12-03T20:45:00-09:00\",\n                \"ends\": \"2025-12-04T05:00:00-09:00\",\n                \"status\": \"Actual\",\n                \"messageType\": \"Alert\",\n                \"category\": \"Met\",\n                \"severity\": \"Minor\",\n                \"certainty\": \"Likely\",\n                \"urgency\": \"Expected\",\n                \"event\": \"Small Craft Advisory\",\n                \"sender\": \"w-nws.webmaster@noaa.gov\",\n                \"senderName\": \"NWS Juneau AK\",\n                \"headline\": \"Small Craft Advisory issued December 3 at 2:44AM AKST until December 4 at 5:00AM AKST by NWS Juneau AK\",\n                \"description\": \"Coastal Waters Forecast for Yakutat Bay\\n\\nWind forecasts reflect the predominant speed and direction\\nexpected. Sea forecasts represent the average of the highest\\none-third of the combined windwave and swell height.\\n\\n.TODAY...E wind 15 kt becoming SE in the afternoon. Seas 10 ft.\\nRain.\\n.TONIGHT...S wind 10 kt in the evening becoming light. Seas 9 ft.\\nS swell. Rain.\\n.THU...Light winds becoming E 10 kt in the afternoon. Seas\\n8 ft. S swell. Rain.\\n.THU NIGHT...E wind 15 kt. Seas 7 ft. SW swell. Rain.\\n.FRI...E wind 25 kt. Seas 7 ft.\\n.SAT...E gale to 35 kt. Seas 11 ft.\\n.SUN...E gale to 35 kt. Seas 12 ft.\",\n                \"instruction\": null,\n                \"response\": \"Avoid\",\n                \"parameters\": {\n                    \"AWIPSidentifier\": [\n                        \"CWFYAK\"\n                    ],\n                    \"WMOidentifier\": [\n                        \"FZAK53 PAJK 031144\"\n                    ],\n                    \"NWSheadline\": [\n                        \"SMALL CRAFT ADVISORY THROUGH LATE TONIGHT\"\n                    ],\n                    \"BLOCKCHANNEL\": [\n                        \"EAS\",\n                        \"NWEM\",\n                        \"CMAS\"\n                    ],\n                    \"VTEC\": [\n                        \"/O.NEW.PAJK.SC.Y.2572.251203T1100Z-251204T1400Z/\"\n                    ],\n                    \"eventEndingTime\": [\n                        \"2025-12-04T05:00:00-09:00\"\n                    ]\n                },\n                \"scope\": \"Public\",\n                \"code\": \"IPAWSv1.0\",\n                \"language\": \"en-US\",\n                \"web\": \"http://www.weather.gov\",\n                \"eventCode\": {\n                    \"SAME\": [\n                        \"NWS\"\n                    ],\n                    \"NationalWeatherService\": [\n                        \"SCY\"\n                    ]\n                }\n            }\n        },\n        {\n            \"id\": \"https://api.weather.gov/alerts/urn:oid:2.49.0.1.840.0.eda6a12a51dab3b83bf60aa6decb3c42e9ebbac9.001.1\",\n            \"type\": \"Feature\",\n            \"geometry\": null,\n            \"properties\": {\n                \"@id\": \"https://api.weather.gov/alerts/urn:oid:2.49.0.1.840.0.eda6a12a51dab3b83bf60aa6decb3c42e9ebbac9.001.1\",\n                \"@type\": \"wx:Alert\",\n                \"id\": \"urn:oid:2.49.0.1.840.0.eda6a12a51dab3b83bf60aa6decb3c42e9ebbac9.001.1\",\n                \"areaDesc\": \"Moriches Inlet NY to Montauk Point NY out 20 nm; Fire Island Inlet NY to Moriches Inlet NY out 20 nm\",\n                \"geocode\": {\n                    \"SAME\": [\n                        \"073350\",\n                        \"073353\"\n                    ],\n                    \"UGC\": [\n                        \"ANZ350\",\n                        \"ANZ353\"\n                    ]\n                },\n                \"affectedZones\": [\n                    \"https://api.weather.gov/zones/forecast/ANZ350\",\n                    \"https://api.weather.gov/zones/forecast/ANZ353\"\n                ],\n                \"references\": [\n                    {\n                        \"@id\": \"https://api.weather.gov/alerts/urn:oid:2.49.0.1.840.0.65e698b6ba470dcf13b408ab2bfb144a0f90de6e.001.1\",\n                        \"identifier\": \"urn:oid:2.49.0.1.840.0.65e698b6ba470dcf13b408ab2bfb144a0f90de6e.001.1\",\n                        \"sender\": \"w-nws.webmaster@noaa.gov\",\n                        \"sent\": \"2025-12-03T03:02:00-05:00\"\n                    }\n                ],\n                \"sent\": \"2025-12-03T06:40:00-05:00\",\n                \"effective\": \"2025-12-03T06:40:00-05:00\",\n                \"onset\": \"2025-12-03T06:40:00-05:00\",\n                \"expires\": \"2025-12-03T19:45:00-05:00\",\n                \"ends\": \"2025-12-04T15:00:00-05:00\",\n                \"status\": \"Actual\",\n                \"messageType\": \"Update\",\n                \"category\": \"Met\",\n                \"severity\": \"Minor\",\n                \"certainty\": \"Likely\",\n                \"urgency\": \"Expected\",\n                \"event\": \"Small Craft Advisory\",\n                \"sender\": \"w-nws.webmaster@noaa.gov\",\n                \"senderName\": \"NWS Upton NY\",\n                \"headline\": \"Small Craft Advisory issued December 3 at 6:40AM EST until December 4 at 3:00PM EST by NWS Upton NY\",\n                \"description\": \"* WHAT...For the Small Craft Advisory, west winds 15 to 20 kt with\\ngusts up to 25 kt and seas 4 to 7 feet. For the Gale Watch,\\nnorthwest winds 20 to 30 kt with gusts up to 40 kt and seas 5 to\\n8 feet possible.\\n\\n* WHERE...Fire Island Inlet NY to Montauk Point NY out 20 nm.\\n\\n* WHEN...For the Small Craft Advisory, until 3 PM EST Thursday.\\nFor the Gale Watch, from Thursday afternoon through late\\nThursday night.\\n\\n* IMPACTS...Strong winds can cause hazardous seas which could\\ncapsize or damage vessels and reduce visibility.\",\n                \"instruction\": \"Mariners should consider altering plans to avoid possible\\nhazardous conditions.  Remain in port, seek safe harbor, alter\\ncourse, and/or secure the vessel for severe wind and seas.\",\n                \"response\": \"Avoid\",\n                \"parameters\": {\n                    \"AWIPSidentifier\": [\n                        \"MWWOKX\"\n                    ],\n                    \"WMOidentifier\": [\n                        \"WHUS71 KOKX 031140\"\n                    ],\n                    \"NWSheadline\": [\n                        \"SMALL CRAFT ADVISORY REMAINS IN EFFECT UNTIL 3 PM EST THURSDAY... ...GALE WATCH REMAINS IN EFFECT FROM THURSDAY AFTERNOON THROUGH LATE THURSDAY NIGHT\"\n                    ],\n                    \"BLOCKCHANNEL\": [\n                        \"EAS\",\n                        \"NWEM\",\n                        \"CMAS\"\n                    ],\n                    \"VTEC\": [\n                        \"/O.CON.KOKX.SC.Y.0111.000000T0000Z-251204T2000Z/\"\n                    ],\n                    \"eventEndingTime\": [\n                        \"2025-12-04T15:00:00-05:00\"\n                    ],\n                    \"expiredReferences\": [\n                        \"w-nws.webmaster@noaa.gov,urn:oid:2.49.0.1.840.0.ccba0ca9284c1e638a678cfbb9d4c4131fa82910.001.1,2025-12-02T13:01:00-05:00 w-nws.webmaster@noaa.gov,urn:oid:2.49.0.1.840.0.f66193c09c556463d3d8c63bce1b034f3b0ce6c5.001.1,2025-12-02T01:36:00-05:00 w-nws.webmaster@noaa.gov,urn:oid:2.49.0.1.840.0.57e44e37368416f721b2e96097448da44f0e554e.001.2,2025-12-01T13:22:00-05:00\"\n                    ]\n                },\n                \"scope\": \"Public\",\n                \"code\": \"IPAWSv1.0\",\n                \"language\": \"en-US\",\n                \"web\": \"http://www.weather.gov\",\n                \"eventCode\": {\n                    \"SAME\": [\n                        \"NWS\"\n                    ],\n                    \"NationalWeatherService\": [\n                        \"SCY\"\n                    ]\n                }\n            }\n        },\n        {\n            \"id\": \"https://api.weather.gov/alerts/urn:oid:2.49.0.1.840.0.eda6a12a51dab3b83bf60aa6decb3c42e9ebbac9.002.1\",\n            \"type\": \"Feature\",\n            \"geometry\": null,\n            \"properties\": {\n                \"@id\": \"https://api.weather.gov/alerts/urn:oid:2.49.0.1.840.0.eda6a12a51dab3b83bf60aa6decb3c42e9ebbac9.002.1\",\n                \"@type\": \"wx:Alert\",\n                \"id\": \"urn:oid:2.49.0.1.840.0.eda6a12a51dab3b83bf60aa6decb3c42e9ebbac9.002.1\",\n                \"areaDesc\": \"Sandy Hook NJ to Fire Island Inlet NY out 20 nm\",\n                \"geocode\": {\n                    \"SAME\": [\n        
